vi "runViWithOutput.vi"(8 "error in (no error)":errorcluster, 10 "vi path":path, 11 "SalProcess in":refnum<class "SalProcess.lvclass">) -> (0 "error out":errorcluster, 1 "function return":i32, 2 "variant":variant, 3 "SalProcess out":refnum<class "SalProcess.lvclass">)   [LabVIEW 2018, in "SalProcess.lvclass"]
doc: "Run the vi with outputs."
uses:
  SalProcess.lvclass
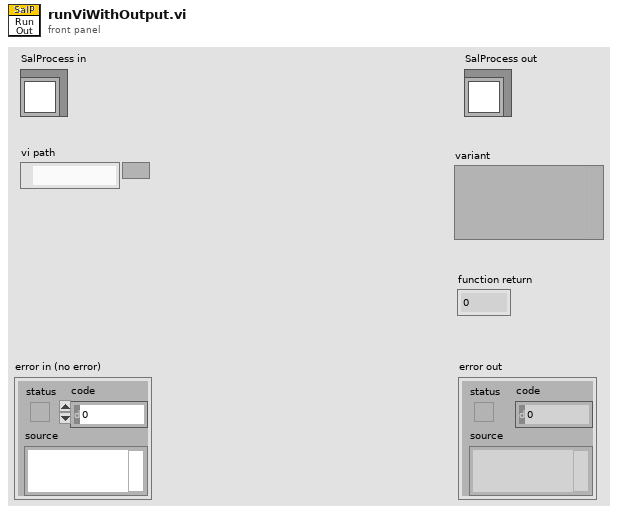
[diagram p1: front panel]
types:
  T1 = typedef "SALLV_Test.lvlib/logevent_summaryState.ctl" = cluster{"private_rcvStamp":dbl, "summaryState":enum32{"", "DisabledState", "EnabledState", "FaultState", "OfflineState", "StandbyState"}, "priority":i32}
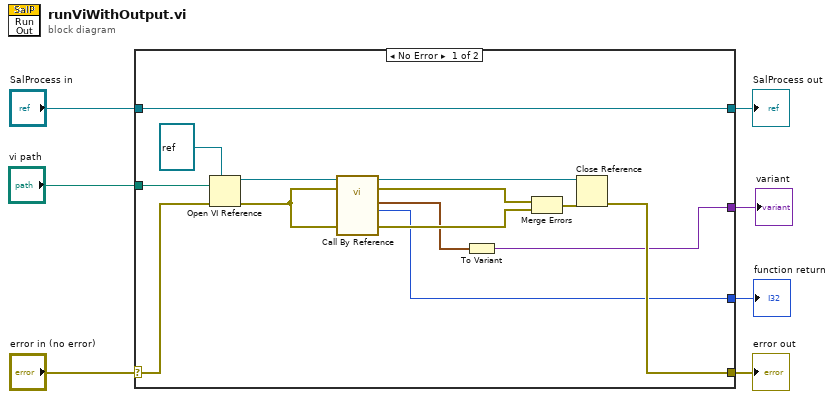
[diagram p0: block diagram]
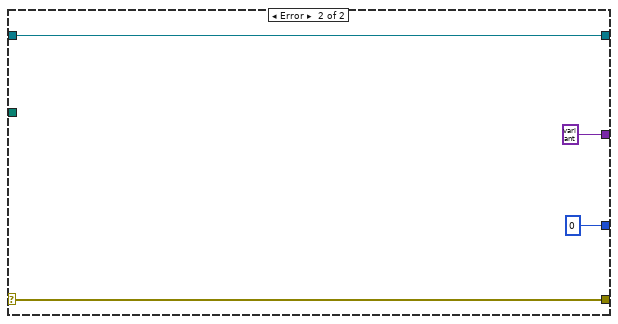
[diagram p2: hidden frame]
diagram:
  n1 = case shown="No Error" "error in (no error)" {
    selector: "error in (no error)" -> [w19 w25]
    tunnel: [w13 w25] -> w6
    tunnel: [w21 w24] -> w4
    tunnel: "SalProcess in" -> [w21 w24]
    tunnel: "vi path" -> [w20 _]
    tunnel: [w12 0 ("function return")] -> w2
    tunnel: [w8 variant ("Variant")] -> w1
    frame No Error {
      n2 = Open VI Reference(type specifier VI Refnum (for type only)=refnum<vi> refnum, vi path=w20, error in (no error)=w19) -> (vi reference=w10:refnum<vi>, error out=w11:errorcluster)  [unwired: 3 in]
      n3 = call-by-ref "?"(reference=w10, error in=w11, 8:"error in (no error)"=w11) -> (reference out=w17:refnum<vi>, error out=w16:errorcluster, 0:"error out"=w15:errorcluster, "function return"=w12:i32, "logevent_summaryState_Ctl out"=w9:T1)  [unwired: 8 in]
      n4 = To Variant(anything=w9) -> (Variant=w8:variant)
      n5 = Merge Errors(w16, w15) -> (w14:errorcluster)
      n6 = Close Reference(reference=w17, error in (no error)=w14) -> (error out=w13:errorcluster)
    }
    frame Error {
    }
  }
  "error out" <- w6
  "SalProcess out" <- w4
  "variant" <- w1
  "function return" <- w2
